vi "XY8-N.vi"(0 "Tau":dbl[unit]=1e-08 format="%#_13g", 1 "Gain":dbl=0.65 format="%#_13g", 2 "MW switch margin (ns)":dbl=30.0 format="%#_13g", 3 "resolution (ns)":dbl=0.5 format="%#_13g", 5 "pi":dbl[unit]=6.5e-09 format="%#_13g", 9 "pi/2":dbl[unit]=3.0000000000000004e-09 format="%#_13g", 11 "margin (ns)":dbl=10.0 format="%#_13g", 12 "AOM on":dbl[unit]=9.999999999999999e-06 format="%#_13g", 13 "AOM off":dbl[unit]=5e-07 format="%#_13g", 14 "N":i32=1) -> (4 "Array size":dbl=25000.0 format="%#_13g", 6 "I array":dbl[](array[numeric]), 10 "Q array":dbl[](array[numeric]), 15 "pulse length (ns)":dbl=238.0)   [LabVIEW 2015]
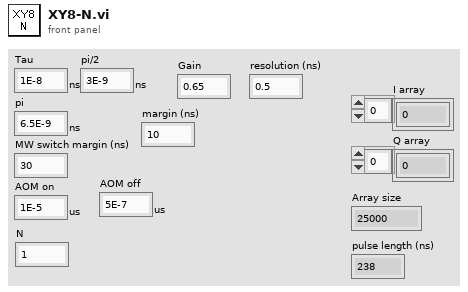
[diagram p1: front panel]
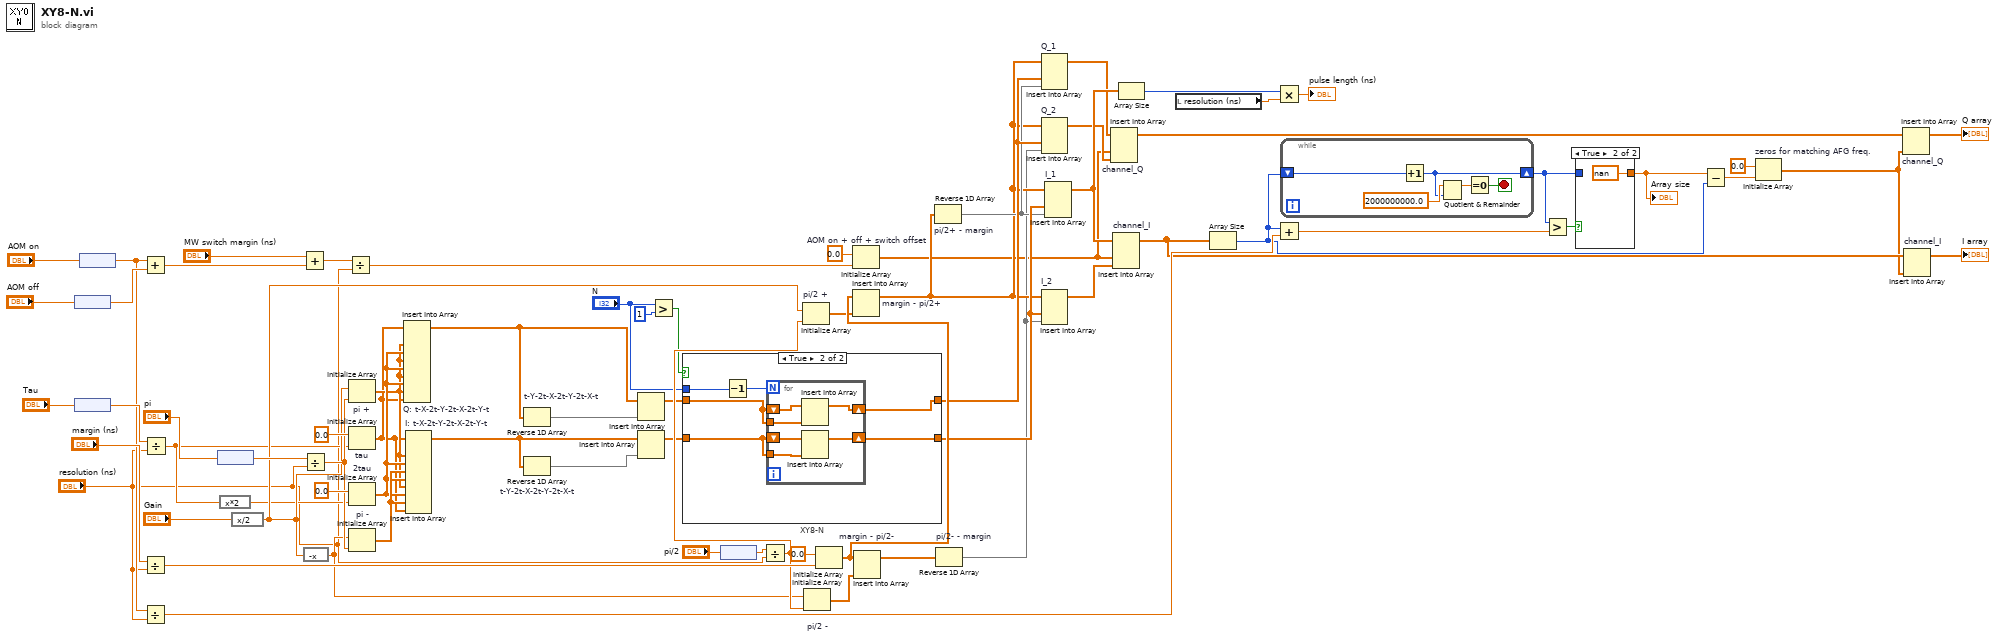
[diagram p0: block diagram]
diagram:
  n1 = node("AOM off") -> (w30:dbl)
  n2 = node("Tau") -> (w57:dbl)
  n3 = node("AOM on") -> (w28:dbl)
  n4 = Add(x=w28, y=w30) -> (x+y=w29:dbl)
  n5 = Divide(x="margin (ns)", y="resolution (ns)") -> (x/y=w69:dbl)
  n6 = Divide(x=w28, y="resolution (ns)") -> (x/y=w25:dbl)
  n7 = Divide(x=w57, y="resolution (ns)") -> (x/y=w45:dbl)
  n8 = node("pi") -> (w58:dbl)
  n9 = expression code="x*2"(w45) -> (w46:dbl)
  n10 = expression code="x/2"("Gain") -> (w53:dbl)
  n11 = Add(x="MW switch margin (ns)", y=w29) -> (x+y=w50:dbl)
  n12 = Divide(x=w58, y="resolution (ns)") -> (x/y=w54:dbl)
  n13 = expression code="-x"(w53) -> (w52:dbl)
  n14 = Divide(x=w50, y="resolution (ns)") -> (x/y=w49:dbl)
  n15 = Initialize Array "pi +"(w53, w54) -> (w34:dbl[])
  n16 = Initialize Array "tau"(0.0 ("element"), w45) -> (w33:dbl[])
  n17 = Initialize Array "2tau"(0.0 ("element"), w46) -> (w35:dbl[])
  n18 = Initialize Array "pi -"(w52, w54) -> (w47:dbl[])
  n19 = Insert Into Array "Q: t-X-2t-Y-2t-X-2t-Y-t"(array=w33, new element #1=w34, new element #2=w35, new element #3=w34, new element #4=w35, new element #5=w34, new element #6=w35, new element #7=w34, new element #8=w33) -> (w37:dbl[])  [unwired: 1 in]
  n20 = Insert Into Array "I: t-X-2t-Y-2t-X-2t-Y-t"(array=w33, new element #1=w34, new element #2=w35, new element #3=w47, new element #4=w35, new element #5=w34, new element #6=w35, new element #7=w47, new element #8=w33) -> (w44:dbl[])  [unwired: 1 in]
  n21 = Reverse 1D Array "t-Y-2t-X-2t-Y-2t-X-t"(array=w37) -> (reversed array=w38:dbl[])
  n22 = Reverse 1D Array "t-Y-2t-X-2t-Y-2t-X-t"(array=w44) -> (reversed array=w43:dbl[])
  n23 = Insert Into Array(array=w37, new element=w38) -> (w36:dbl[])  [unwired: 1 in]
  n24 = Insert Into Array(array=w44, new element=w43) -> (w42:dbl[])  [unwired: 1 in]
  n25 = Greater?(x="N", y=1) -> (0:w39:bool)
  n26 = case "XY8-N" shown="True" w39 {
    tunnel: "N" -> [_ w78]
    tunnel: w42 -> [w73 w76]
    tunnel: [w73 w79] -> w14
    tunnel: w36 -> [w72 w75]
    tunnel: [w72 w74] -> w8
    frame False {
    }
    frame True {
      n27 = Decrement(x=w78) -> (x-1=w77:i32)
      n28 = for {
        N: w77 -> [_]
        shift-right: [w85] -> w79
        shift-left: w76 -> [w84]
        tunnel: w76 -> [w83]
        shift-right: [w82] -> w74
        shift-left: w75 -> [w81]
        tunnel: w75 -> [w80]
        n29 = Insert Into Array(array=w81, new element=w80) -> (w82:dbl[])  [unwired: 1 in]
        n30 = Insert Into Array(array=w84, new element=w83) -> (w85:dbl[])  [unwired: 1 in]
      }
    }
  }
  n31 = node("pi/2") -> (w66:dbl)
  n32 = Divide(x=w66, y="resolution (ns)") -> (x/y=w65:dbl)
  n33 = Initialize Array "pi/2 +"(w53, w65) -> (w63:dbl[])
  n34 = Initialize Array "pi/2 -"(w52, w65) -> (w62:dbl[])
  n35 = Initialize Array(0.0 ("element"), w69) -> (w64:dbl[])
  n36 = Initialize Array "AOM on + off + switch offset"(0.0 ("element"), w49) -> (w2:dbl[])
  n37 = Insert Into Array "margin - pi/2+"(array=w64, new element=w63) -> (w6:dbl[])  [unwired: 1 in]
  n38 = Insert Into Array "margin - pi/2-"(array=w64, new element=w62) -> (w61:dbl[])  [unwired: 1 in]
  n39 = Reverse 1D Array "pi/2+ - margin"(array=w6) -> (reversed array=w7:dbl[])
  n40 = Reverse 1D Array "pi/2- - margin"(array=w61) -> (reversed array=w5:dbl[])
  n41 = Insert Into Array "Q_1"(array=w6, new element #1=w8, new element #2=w7) -> (w3:dbl[])  [unwired: 1 in]
  n42 = Insert Into Array "Q_2"(array=w6, new element #1=w8, new element #2=w5) -> (w4:dbl[])  [unwired: 1 in]
  n43 = Insert Into Array "I_2"(array=w6, new element #1=w14, new element #2=w5) -> (w13:dbl[])  [unwired: 1 in]
  n44 = Insert Into Array "I_1"(array=w6, new element #1=w14, new element #2=w7) -> (w12:dbl[])  [unwired: 1 in]
  n45 = Insert Into Array "channel_Q"(array=w3, new element #1=w2, new element #2=w4) -> (w1:dbl[])  [unwired: 1 in]
  n46 = Insert Into Array "channel_I"(array=w12, new element #1=w2, new element #2=w13) -> (w22:dbl[])  [unwired: 1 in]
  n47 = Array Size(array=w12) -> (size(s)=w11:i32)
  n48 = local read "resolution (ns)"() -> (w10:dbl)
  n49 = Array Size(array=w22) -> (size(s)=w20:i32)
  n50 = Multiply(x=w11, y=w10) -> (x*y=→"pulse length (ns)":dbl)
  n51 = Add(x=w20, y=w25) -> (x+y=w26:dbl)
  n52 = while {
    shift-right: [w87] -> w23
    shift-left: w20 -> [w88]
    stop <- w86 stop-if-true
    n53 = Increment(x=w88) -> (x+1=w87:i32)
    n54 = Quotient & Remainder(x=2000000000.0, y=w87) -> (x-y*floor(x/y)=w89:dbl)  [unwired: 1 out]
    n55 = Equal To 0?(x=w89) -> (x = 0?=w86:bool)
  }
  n56 = Greater?(x=w23, y=w26) -> (0:w24:bool)
  n57 = case shown="True" w24 {
    tunnel: [w91 nan] -> w21
    tunnel: w23 -> [w91 _]
    frame False {
    }
    frame True {
    }
  }
  "Array size" <- w21
  n58 = Subtract(x=w21, y=w20) -> (x-y=w19:dbl)
  n59 = Initialize Array "zeros for matching AFG freq."(0.0 ("element"), w19) -> (w17:dbl[])
  n60 = Insert Into Array "channel_Q"(array=w1, new element=w17) -> (→"Q array":dbl[])  [unwired: 1 in]
  n61 = Insert Into Array "channel_I"(array=w22, new element=w17) -> (→"I array":dbl[])  [unwired: 1 in]
